vi "test_mp3.vi"() -> ()   [LabVIEW 2010]
uses:
  <vilib>/measure/NI_MABase.lvlib
panel:
  out "error out":errorcluster
  out "Waveform Graph":waveform(dbl)[](graph)
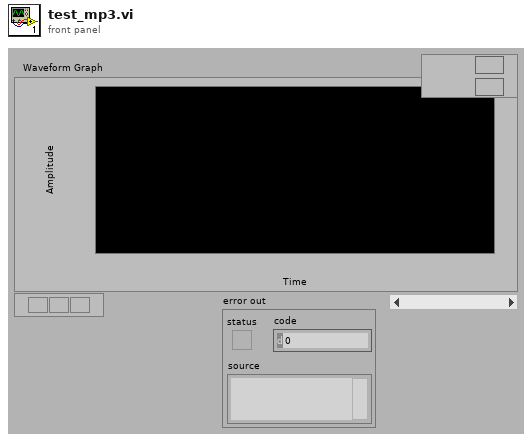
[diagram p1: front panel]
types:
  T1 = enum16{"Sine Wave", "Triangle Wave", "Square Wave", "Sawtooth Wave"}[]
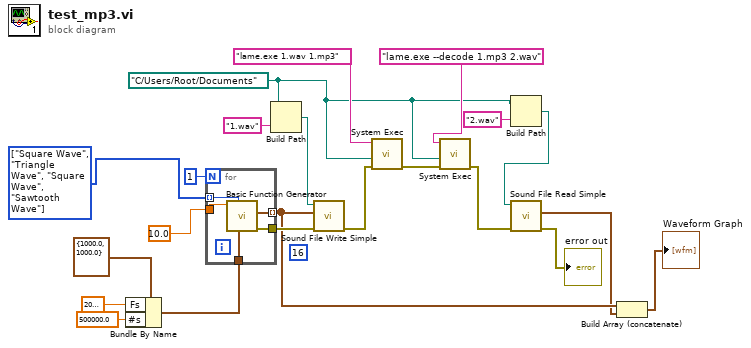
[diagram p0: block diagram]
diagram:
  w16 = T1 [enum."Square Wave", enum."Triangle Wave", enum."Square Wave", enum."Sawtooth Wave"] items=["Sine Wave", "Triangle Wave", "Square Wave", "Sawtooth Wave"]
  (unwired) 16 ("bits per sample")
  w6 = path "C:/Users/Root/Documents" ("path")
  n1 = Bundle By Name(cluster=cluster{"Fs":dbl, "#s":dbl} {"Fs"=1000.0, "#s"=1000.0} ("sampling info"), "Fs"=20000.0 ("#s"), "#s"=500000.0) -> (w18:cluster{"Fs":dbl, "#s":dbl})
  n2 = for {
    N: 1 -> [_]
    tunnel: [w27] -> w22
    tunnel: w16 -> [w26] mode=indexing
    tunnel: w18 -> [w25]
    tunnel: 10.0 ("frequency") -> [w24]
    tunnel: [w23] -> w3 mode=indexing
    n3 = call <vilib>:"Basic Function Generator.vi"("sampling info"=w25, "signal type"=w26, "frequency"=w24) -> ("error out"=w27:errorcluster, "signal out"=w23:waveform(dbl))  [unwired: 6 in, 1 out]
  }
  n4 = Build Path(base path=w6, name or relative path="1.wav") -> (appended path=w11:path)
  n5 = call <vilib>:"Sound File Write Simple.vi"("error in (no error)"=w22, "data"=w3, "path"=w11) -> ("error out"=w13:errorcluster)  [unwired: 7 in, 1 out]
  n6 = call <vilib>:"System Exec.vi"("error in (no error)"=w13, "working directory"=w6, "command line"="lame.exe 1.wav 1.mp3") -> ("error out"=w9:errorcluster)  [unwired: 5 in, 3 out]
  n7 = call <vilib>:"System Exec.vi"("error in (no error)"=w9, "working directory"=w6, "command line"="lame.exe --decode 1.mp3 2.wav") -> ("error out"=w8:errorcluster)  [unwired: 5 in, 3 out]
  n8 = Build Path(base path=w6, name or relative path="2.wav") -> (appended path=w5:path)
  n9 = call <vilib>:"Sound File Read Simple.vi"("error in (no error)"=w8, "path"=w5) -> ("error out"=→"error out":errorcluster, "data"=w2:waveform(dbl)[])  [unwired: 6 in, 2 out]
  n10 = Build Array (concatenate)(w3, w2) -> (→"Waveform Graph":waveform(dbl)[])
